vi "wielomiany.vi"() -> ()   [LabVIEW 2023]
panel:
  in  "Boolean":bool
  in  "stop":bool
  out "y":string
  in  "Enum":T1(ring)
  in  "c":dbl
  in  "b":dbl
  in  "a":dbl
  in  "x":dbl
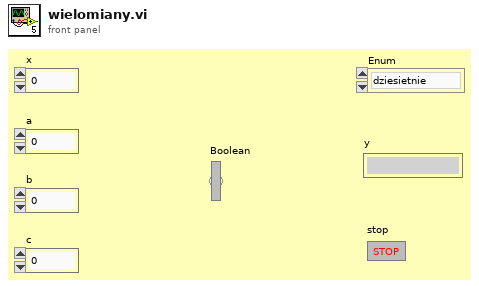
[diagram p1: front panel]
types:
  T1 = enum16{"dziesietnie", "szesnastkowo", "ósemkowo"}
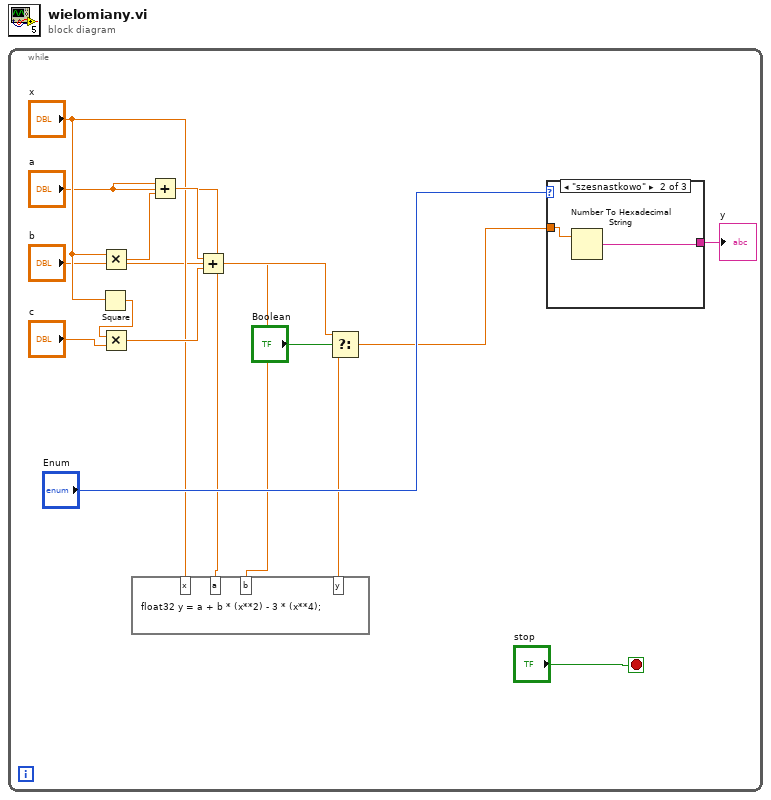
[diagram p0: block diagram]
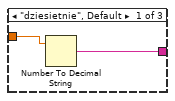
[diagram p2: hidden frame]
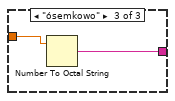
[diagram p3: hidden frame]
diagram:
  n1 = while {
    stop <- "stop" stop-if-true
    n2 = Square(x="x") -> (x^2=w13:dbl)
    n3 = Multiply(x="x", y="b") -> (x*y=w15:dbl)
    n4 = Multiply(x=w13, y="c") -> (x*y=w12:dbl)
    n5 = formula code="float32 y = a + b * (x**2) - 3 * (x**4);"("x"="x", "a"="a", "b"="b") -> ("y"=w5:sgl)
    n6 = Add(x="a", y=w15) -> (x+y=w11:dbl)
    n7 = Add(x=w11, y=w12) -> (x+y=w6:dbl)
    n8 = Select(t=w6, s="Boolean", f=w5) -> (s? t:f=w4:dbl)
    n9 = case shown="\"szesnastkowo\"" "Enum" {
      tunnel: [w17 w19 w21] -> w8
      tunnel: w4 -> [w16 w18 w20]
      frame "dziesietnie", Default {
        n10 = Number To Decimal String(number=w16) -> (decimal integer string=w17:string)  [unwired: 1 in]
      }
      frame "szesnastkowo" {
        n11 = Number To Hexadecimal String(2:w18) -> (0:w19:string)  [unwired: 1 in]
      }
      frame "ósemkowo" {
        n12 = Number To Octal String(2:w20) -> (0:w21:string)  [unwired: 1 in]
      }
    }
    "y" <- w8
  }
